vi "_AddAfter.vi"(9 "Data":variant, 10 "ID":variant, 11 "Next States in":T1) -> (3 "Next States out":T1)   [LabVIEW 2020]
uses:
  TDefs/States.ctl
  TDefs/State.ctl
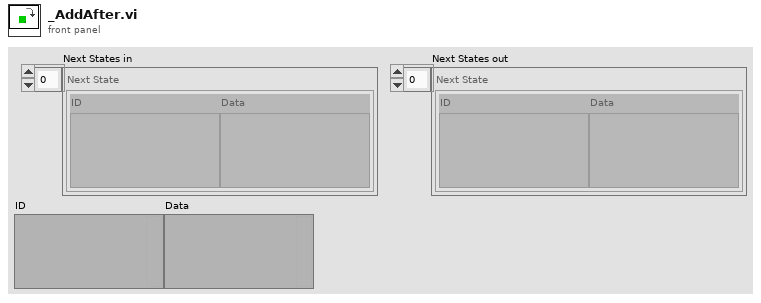
[diagram p1: front panel]
types:
  T1 = typedef "States.ctl" = T2[]
  T2 = typedef "State.ctl" = cluster{"ID":variant, "Data":variant}
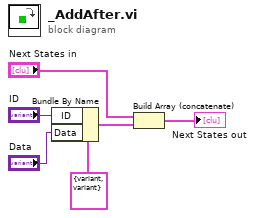
[diagram p0: block diagram]
diagram:
  n1 = Bundle By Name(cluster=T2 {"ID"=variant, "Data"=variant} ("State"), "ID"="ID", "Data"="Data") -> (w5:T2)
  n2 = Build Array (concatenate)("Next States in", w5) -> (→"Next States out":T1)
